vi "ex_Wire Con Pane.vi"(8 "error in (no error)":errorcluster, 9 "All Controls":string[](array[string]), 10 "Controls to Wire":string[](array[string]), 11 "VI refnum":refnum<vi>) -> (0 "Error Out":errorcluster, 2 "Controls[]":refnum<vi>[](array[refnum]), 3 "VI refnum out":refnum<vi>)   [LabVIEW 2020]
doc: "Wires the specified controls on a VI to the connector pane."
panel:
  in  "Array of refnums in":refnum<vi>[](array[refnum])
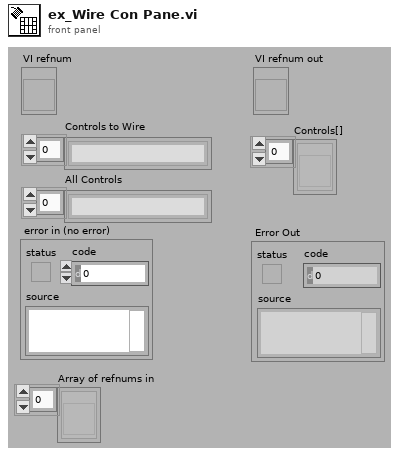
[diagram p1: front panel]
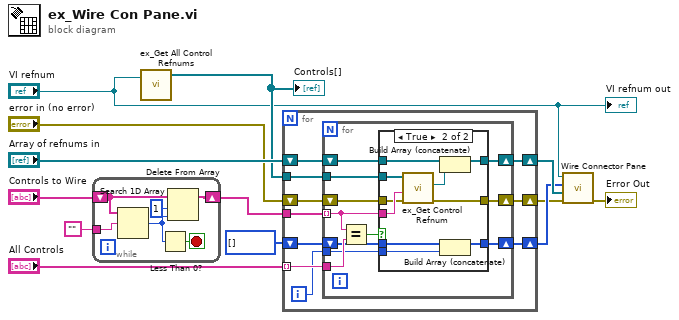
[diagram p0: block diagram]
diagram:
  n1 = while {
    shift-right: [w17] -> w4
    shift-left: "Controls to Wire" -> [w18]
    tunnel: "" -> [w19]
    stop <- w16 stop-if-true
    n2 = Search 1D Array(1D array=w18, element=w19) -> (index of element=w15:i32)  [unwired: 1 in]
    n3 = Less Than 0?(x=w15) -> (x < 0?=w16:bool)
    n4 = Delete From Array(array=w18, length=1, index=w15) -> (array with subset deleted=w17:string[])  [unwired: 1 out]
  }
  n5 = call <vilib>:"ex_Get All Control Refnums.vi"("viref Express VI"="VI refnum") -> ("All Controls[]"=w3:refnum<vi>[])  [unwired: 2 in, 1 out]
  "Controls[]" <- w3
  n6 = for {
    tunnel: w3 -> [w27]
    tunnel: w4 -> [w28]
    tunnel: "All Controls" -> [w29] mode=indexing
    shift-right: [w20] -> w13
    shift-left: "Array of refnums in" -> [w21]
    shift-right: [w22] -> w12
    shift-left: i32[] [] -> [w23]
    shift-right: [w24] -> w11
    shift-left: "error in (no error)" -> [w25]
    i -> [w26]
    n7 = for {
      tunnel: w29 -> [w40]
      tunnel: w28 -> [w37] mode=indexing
      tunnel: w27 -> [w38]
      tunnel: w26 -> [w36]
      shift-right: [w35] -> w24
      shift-left: w25 -> [w34]
      shift-right: [w33] -> w22
      shift-left: w23 -> [w32]
      shift-right: [w31] -> w20
      shift-left: w21 -> [w30]
      n8 = Equal?(x=w37, y=w40) -> (x = y?=w39:bool)
      n9 = case shown="True" w39 {
        tunnel: w38 -> [_ w53]
        tunnel: w37 -> [_ w52]
        tunnel: [w43 w50] -> w31
        tunnel: w30 -> [w43 w49]
        tunnel: w32 -> [w42 w48]
        tunnel: [w42 w47] -> w33
        tunnel: w36 -> [_ w46]
        tunnel: [w41 w45] -> w35
        tunnel: w34 -> [w41 w44]
        frame False {
        }
        frame True {
          n10 = call <vilib>:"ex_Get Control Refnum.vi"("error in (no error)"=w44, "Name"=w52, "Controls[]"=w53) -> ("error out"=w45:errorcluster, "Ctl Refnum"=w51:refnum<vi>)  [unwired: 7 in]
          n11 = Build Array (concatenate)(w49, w51) -> (w50:refnum<vi>[])
          n12 = Build Array (concatenate)(w48, w46) -> (w47:i32[])
        }
      }
    }
  }
  n13 = call <vilib>:"Wire Connector Pane.vi"("Error In"=w11, "Controls"=w13, "Control Indices"=w12, "VI refnum"="VI refnum") -> ("Error Out"=→"Error Out":errorcluster)  [unwired: 7 in]
  "VI refnum out" <- "VI refnum"
